vi "UpdateMessage (SubVI).vi"(8 "Error In":errorcluster, 11 "UpdateMessageControl":T1={"Command"=enum."Welcome", "Data"=variant}) -> (0 "Error Out":errorcluster, 2 "ATM Messages":T3)   [LabVIEW 2017]
doc: "Outputs a string message depending on the command."
uses:
  Controls/Control 1.ctl
  Controls/UpdateMessageControl.ctl
  Controls/UpdateMessageCommand.ctl
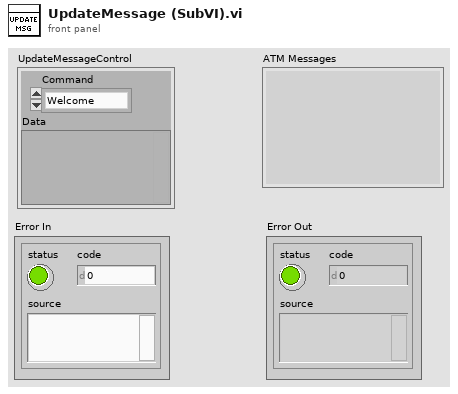
[diagram p1: front panel]
types:
  T1 = typedef "UpdateMessageControl.ctl" = cluster{"Command":T2, "Data":variant}
  T2 = typedef "UpdateMessageCommand.ctl" = enum16{"SystemCrash2", "SystemCrash1", "Welcome", "MainMenu", "PhoneNumberFailed", "PhoneNumberSuccess", "ParcelNumberSuccess", "ParcelNumbertFailed", "SessionTerminate", "SessionFinished", "Deposit", "DepositComplete", "Withdrawal", "WithdrawalComplete", "WithdrawalFailed"}
  T3 = typedef "Control 1.ctl" = string
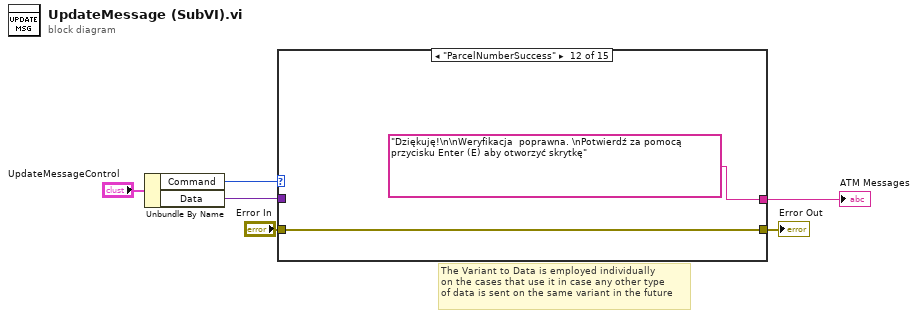
[diagram p0: block diagram]
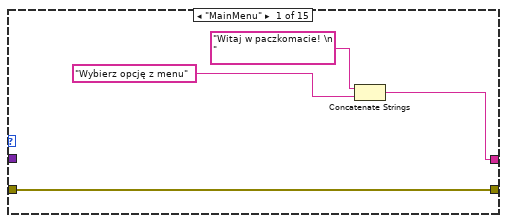
[diagram p2: hidden frame]
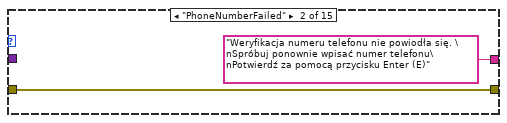
[diagram p3: hidden frame]
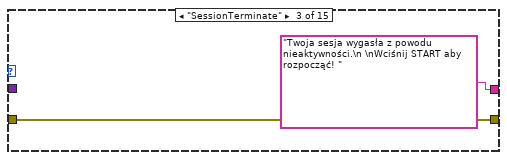
[diagram p4: hidden frame]
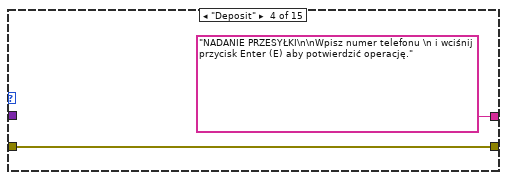
[diagram p5: hidden frame]
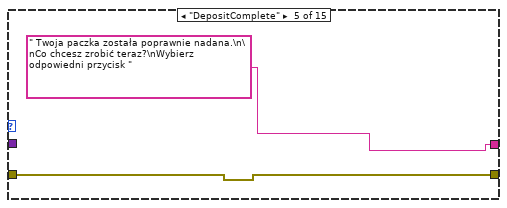
[diagram p6: hidden frame]
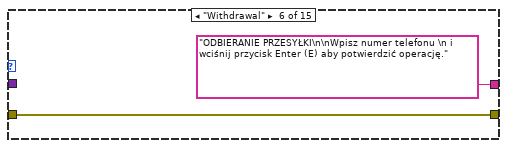
[diagram p7: hidden frame]
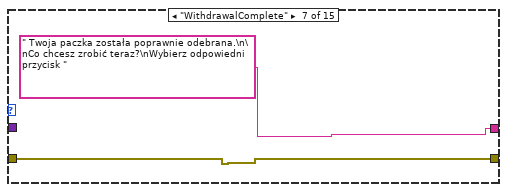
[diagram p8: hidden frame]
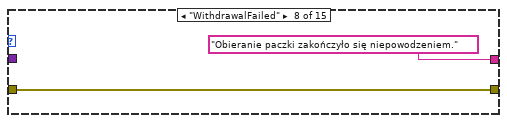
[diagram p9: hidden frame]
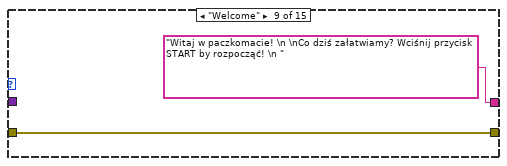
[diagram p10: hidden frame]
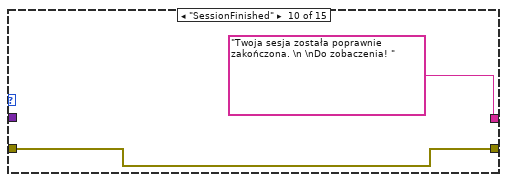
[diagram p11: hidden frame]
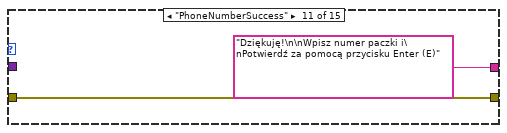
[diagram p12: hidden frame]
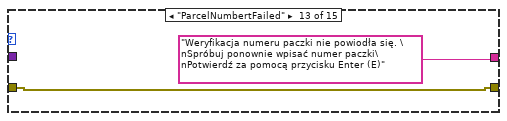
[diagram p13: hidden frame]
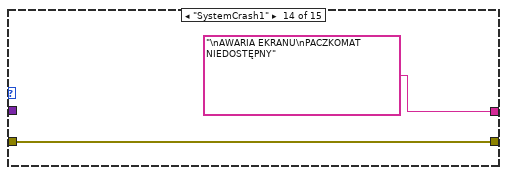
[diagram p14: hidden frame]
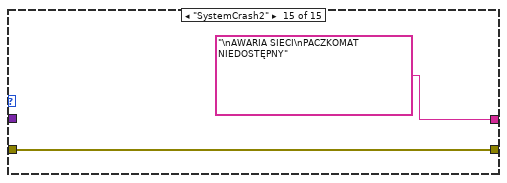
[diagram p15: hidden frame]
diagram:
  # "The Variant to Data is employed individually\non the cases that use it in case any other type\nof data is sent on the same variant in the future"
  n1 = Unbundle By Name("UpdateMessageControl") -> ("Command"=w5:T2, "Data"=w3:variant)
  n2 = case shown="\"ParcelNumberSuccess\"" w5 {
    tunnel: [w9 "Weryfikacja numeru telefonu nie powiodła się. \nSpróbuj ponownie wpisać numer telefonu\nPotwierdź za pomocą przycisku Enter (E)" ("ATM Messages") "Twoja sesja wygasła z powodu nieaktywności.\n \nWciśnij START aby rozpocząć! " ("ATM Messages") "NADANIE PRZESYŁKI\n\nWpisz numer telefonu \n i wciśnij przycisk Enter (E) aby potwierdzić operację." ("ATM Messages") " Twoja paczka została poprawnie nadana.\n\nCo chcesz zrobić teraz?\nWybierz odpowiedni przycisk " ("ATM Messages") "ODBIERANIE PRZESYŁKI\n\nWpisz numer telefonu \n i wciśnij przycisk Enter (E) aby potwierdzić operację." ("ATM Messages") " Twoja paczka została poprawnie odebrana.\n\nCo chcesz zrobić teraz?\nWybierz odpowiedni przycisk " ("ATM Messages") "Obieranie paczki zakończyło się niepowodzeniem." ("ATM Messages") "Witaj w paczkomacie! \n \nCo dziś załatwiamy? Wciśnij przycisk START by rozpocząć! \n " ("ATM Messages") "Twoja sesja została poprawnie zakończona. \n \nDo zobaczenia! " ("ATM Messages") "Dziękuję!\n\nWpisz numer paczki i\nPotwierdź za pomocą przycisku Enter (E)" ("ATM Messages") "Dziękuję!\n\nWeryfikacja  poprawna. \nPotwierdź za pomocą przycisku Enter (E) aby otworzyć skrytkę" ("ATM Messages") "Weryfikacja numeru paczki nie powiodła się. \nSpróbuj ponownie wpisać numer paczki\nPotwierdź za pomocą przycisku Enter (E)" ("ATM Messages") "\nAWARIA EKRANU\nPACZKOMAT NIEDOSTĘPNY" ("ATM Messages") "\nAWARIA SIECI\nPACZKOMAT NIEDOSTĘPNY" ("ATM Messages")] -> w6
    tunnel: w3 -> [_ _ _ _ _ _ _ _ _ _ _ _ _ _ _]
    tunnel: "Error In" -> [w7 w11 w13 w15 w18 w19 w22 w23 w25 w27 w29 w32 w33 w35 w37]
    tunnel: [w7 w11 w13 w15 w18 w19 w22 w23 w25 w27 w29 w32 w33 w35 w37] -> w1
    frame "MainMenu" {
      n3 = Concatenate Strings("Witaj w paczkomacie! \n  " ("ATM Messages"), "Wybierz opcję z menu" ("ATM Messages")) -> (w9:string)
    }
    frame "PhoneNumberFailed" {
    }
    frame "SessionTerminate" {
    }
    frame "Deposit" {
    }
    frame "DepositComplete" {
    }
    frame "Withdrawal" {
    }
    frame "WithdrawalComplete" {
    }
    frame "WithdrawalFailed" {
    }
    frame "Welcome" {
    }
    frame "SessionFinished" {
    }
    frame "PhoneNumberSuccess" {
    }
    frame "ParcelNumberSuccess" {
    }
    frame "ParcelNumbertFailed" {
    }
    frame "SystemCrash1" {
    }
    frame "SystemCrash2" {
    }
  }
  "ATM Messages" <- w6
  "Error Out" <- w1
